vi "Practica5.1_Fórmula Node.vi"() -> ()   [LabVIEW 2022 SP3]
panel:
  out "Area":dbl
  out "Superficie":dbl
  in  "Valor de c":dbl
  in  "Valor de b":dbl
  in  "Valorde a":dbl
  # "Anahí Montserrat Vázquez Padilla \nPráctica 05: Fórmula Node\n13/02/2024"
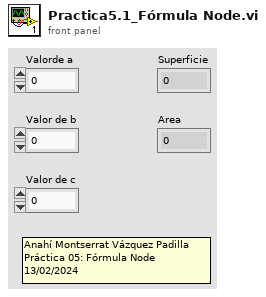
[diagram p1: front panel]
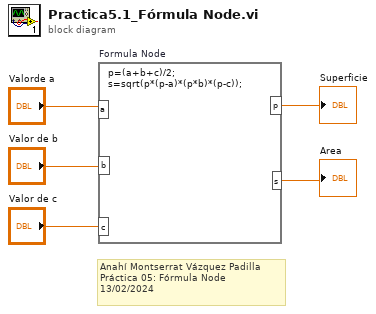
[diagram p0: block diagram]
diagram:
  # "Anahí Montserrat Vázquez Padilla \nPráctica 05: Fórmula Node\n13/02/2024"
  n1 = formula code="p=(a+b+c)/2;\ns=sqrt(p*(p-a)*(p*b)*(p-c));"("a"="Valorde a", "b"="Valor de b", "c"="Valor de c") -> ("p"=→"Superficie":dbl, "s"=→"Area":dbl)
